vi "Read Formatted Default Value.vi"(10 "# of Digits":u8=5, 11 "channel":refnum<class "TBM channel.lvclass">) -> (2 "Formatted Default":string, 3 "channel out":refnum<class "TBM channel.lvclass">)   [LabVIEW 2013]
uses:
  <vilib>/NI/Tag Bus Module Framework/channel/TBM channel.lvclass
  <vilib>/NI/Tag Bus/tag/tag descriptor.lvclass/tag descriptor.ctl
  <vilib>/NI/Tag Bus/tag/read data type.vi
  <vilib>/NI/Tag Bus/tag/tag descriptor.lvclass
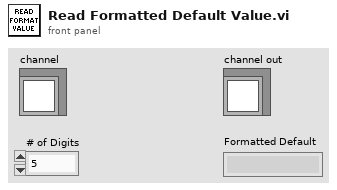
[diagram p1: front panel]
types:
  T1 = typedef "tag bus.lvlib/tag descriptor.lvclass/Data Type.ctl" = enum16{"Double", "Single", "I64", "I32", "I16", "I8", "U64", "U32", "U16", "U8", "Boolean", "String", "Array of Double", "Array of Single", "Array of I64", "Array of I32", "Array of I16", "Array of I8", "Array of U64", "Array of U32", "Array of U16", "Array of U8", "Array of Boolean", "Array of String"}
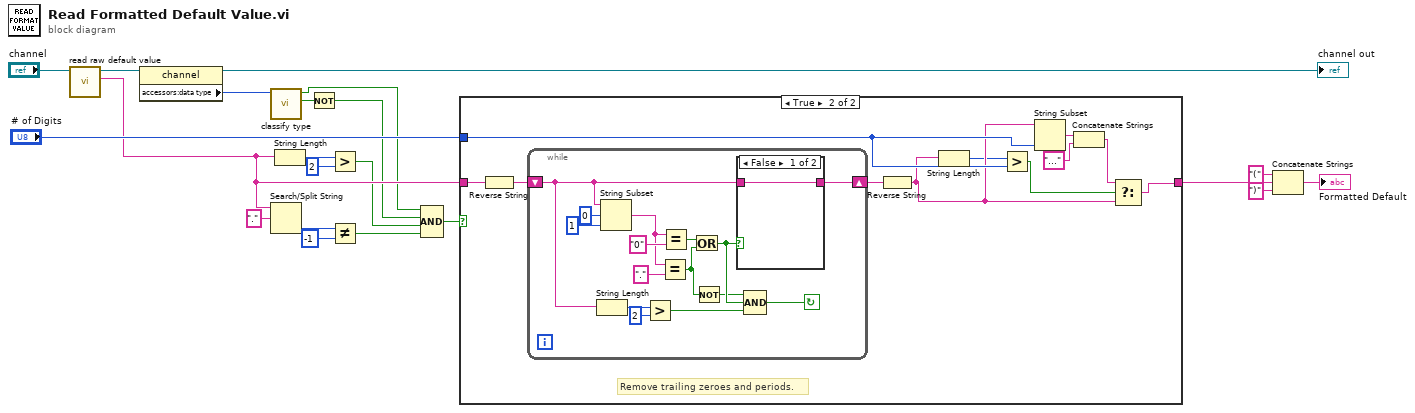
[diagram p0: block diagram]
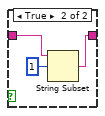
[diagram p3: hidden frame]
diagram:
  n1 = call <vilib>:"read raw default value.vi"("system tag in"="channel") -> ("raw default"=w15:string, "system tag out"=w14:refnum<class "TBM channel.lvclass">)  [unwired: 8 in, 1 out]
  n2 = property class="channel"(reference=w14) -> (reference out=→"channel out":refnum<class "TBM channel.lvclass">, "accessors:data type"=w4:T1)  [unwired: 1 in, 1 out]
  n3 = call <vilib>:"classify type.vi"("data type"=w4) -> ("array?"=w3:bool, "numeric?"=w1:bool)  [unwired: 9 in]
  n4 = Search/Split String(string=w15, search string/char (-)=".") -> (offset of match=w8:i32)  [unwired: 1 in, 2 out]
  n5 = String Length(string=w15) -> (length=w11:i32)
  n6 = Not(x=w3) -> (.not. x?=w2:bool)
  n7 = Greater?(x=w11, y=2) -> (0:w9:bool)
  n8 = Not Equal?(x=w8, y=-1) -> (x != y?=w6:bool)
  n9 = Compound Arithmetic op=AND(w1, w2, w9, w6) -> (w5:bool)
  n10 = case shown="True" w5 {
    tunnel: [w22 w25] -> w16
    tunnel: w15 -> [w22 w31]
    tunnel: "# of Digits" -> [_ w26]
    frame False {
    }
    frame True {
      # "Remove trailing zeroes and periods."
      n11 = Reverse String(1:w31) -> (0:w33:string)
      n12 = while {
        shift-right: [w42] -> w32
        shift-left: w33 -> [w41]
        stop <- w37 continue-if-true
        n13 = String Length(string=w41) -> (length=w40:i32)
        n14 = String Subset(string=w41, offset (0)=0, length (rest)=1 ("length (rest)")) -> (substring=w45:string)
        n15 = Greater?(x=w40, y=2) -> (0:w38:bool)
        n16 = Equal?(x=w45, y=".") -> (x = y?=w36:bool)
        n17 = Equal?(x=w45, y="0") -> (x = y?=w43:bool)
        n18 = Or(x=w43, y=w36) -> (x .or. y?=w35:bool)
        n19 = Not(x=w36) -> (.not. x?=w34:bool)
        n20 = case shown="False" w35 {
          tunnel: w41 -> [w49 w52]
          tunnel: [w49 w50] -> w42
          frame False {
          }
          frame True {
            n21 = String Subset(string=w52, offset (0)=1) -> (substring=w50:string)  [unwired: 1 in]
          }
        }
        n22 = Compound Arithmetic op=AND(w34, w35, w38) -> (w37:bool)
      }
      n23 = Reverse String(1:w32) -> (0:w24:string)
      n24 = String Length(string=w24) -> (length=w23:i32)
      n25 = Greater?(x=w23, y=w26) -> (0:w27:bool)
      n26 = String Subset(string=w24, length (rest)=w26) -> (substring=w29:string)  [unwired: 1 in]
      n27 = Concatenate Strings(w29, "..." ("string")) -> (w28:string)
      n28 = Select(t=w28, s=w27, f=w24) -> (s? t:f=w25:string)
    }
  }
  n29 = Concatenate Strings("(" ("string"), w16, ")" ("string")) -> (→"Formatted Default":string)
